vi "Read Assertion Types.vi"(11 "Conditional Dialog in":refnum<class "Conditional Dialog.lvclass">) -> (2 "Assertion Types":refnum<class "Assert.lvclass">[](array[class]), 3 "Conditional Dialog out":refnum<class "Conditional Dialog.lvclass">)   [LabVIEW 2017, in "Conditional Dialog.lvclass"]
uses:
  Conditional Dialog.lvclass
  <vilib>/gpm_packages/@cs/run-time-assertions/Source/Assert/Assert.lvclass
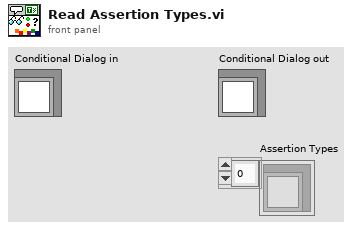
[diagram p1: front panel]
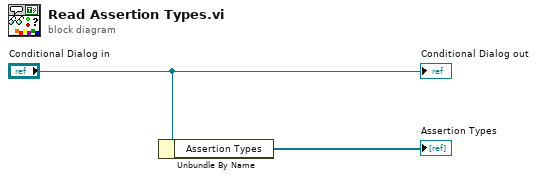
[diagram p0: block diagram]
diagram:
  n1 = Unbundle By Name("Conditional Dialog in") -> ("Assertion Types"=→"Assertion Types":refnum<class "Assert.lvclass">[])
  "Conditional Dialog out" <- "Conditional Dialog in"
